vi "DS11202Z CHx-Config.vi"(0 "TestIndex":i32, 1 "通道":enum16{"Channel_1", "Channel_2"}(ring), 2 "通道开关":enum16{"ON", "OFF"}(ring), 3 "耦合":enum16{"直流", "交流", "接地"}(ring)=enum."接地", 4 "探头":enum16{"1X", "10X"}(ring)=enum."10X", 5 "幅值":dbl=1.0) -> (14 "OK?":bool, 19 "错误输出":errorcluster)   [LabVIEW 2015]
panel:
  out "Command":string
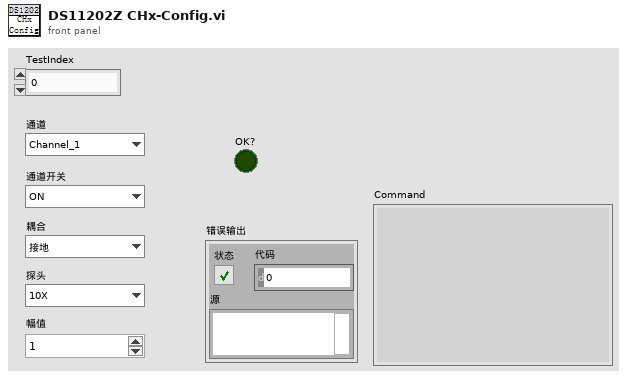
[diagram p1: front panel]
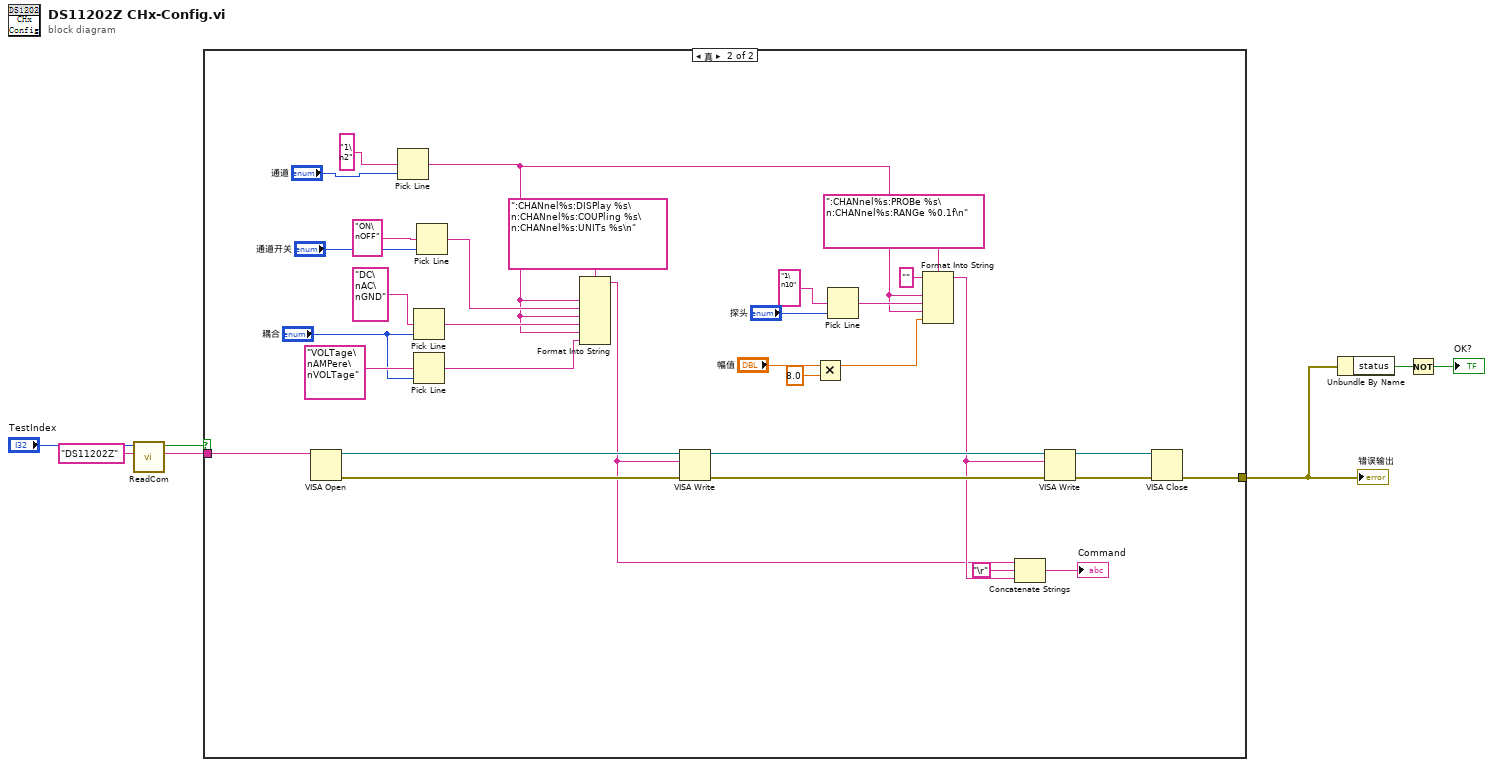
[diagram p0: block diagram]
diagram:
  n1 = call "ReadCom.vi"("仪器名称"="DS11202Z", "MyIndex"="TestIndex") -> ("COM"=w1:string, "OK?"=w2:bool)  [unwired: 7 in, 1 out]
  n2 = case shown="真" w2 {
    tunnel: [_ w34] -> w7
    tunnel: w1 -> [_ w8]
    frame False {
    }
    frame True {
      n3 = VISA Open(VISA resource name=w8) -> (VISA resource name=w39:refnum<visa-resource-name>, error out=w38:errorcluster)  [unwired: 1 in, 3 out]
      n4 = Pick Line(multi-line string="1\n2", line index="通道") -> (output string=w14:string)  [unwired: 1 in]
      n5 = Pick Line(multi-line string="DC\nAC\nGND", line index="耦合") -> (output string=w26:string)  [unwired: 1 in]
      n6 = Pick Line(multi-line string="VOLTage\nAMPere\nVOLTage", line index="耦合") -> (output string=w19:string)  [unwired: 1 in]
      n7 = Pick Line(multi-line string="ON\nOFF", line index="通道开关") -> (output string=w27:string)  [unwired: 1 in]
      n8 = Format Into String(format string=":CHANnel%s:DISPlay %s\n:CHANnel%s:COUPling %s\n:CHANnel%s:UNITs %s\n" ("字符串"), w14, w27, w14, w26, w14, w19) -> (resulting string=w10:string)  [unwired: 2 in, 1 out]
      n9 = VISA Write(VISA resource name=w39, write buffer=w10, error in (no error)=w38) -> (VISA resource name out=w37:refnum<visa-resource-name>, error out=w36:errorcluster)  [unwired: 1 out]
      n10 = Multiply(x="幅值", y=8.0) -> (x*y=w13:dbl)
      n11 = Pick Line(multi-line string="1\n10", line index="探头") -> (output string=w18:string)  [unwired: 1 in]
      n12 = Format Into String(format string=":CHANnel%s:PROBe %s\n:CHANnel%s:RANGe %0.1f\n" ("字符串"), initial string="" ("初始字符串"), w14, w18, w14, w13) -> (resulting string=w35:string)  [unwired: 1 in, 1 out]
      n13 = Concatenate Strings(w10, "\r", w35) -> (→"Command":string)
      n14 = VISA Write(VISA resource name=w37, write buffer=w35, error in (no error)=w36) -> (VISA resource name out=w23:refnum<visa-resource-name>, error out=w22:errorcluster)  [unwired: 1 out]
      n15 = VISA Close(VISA resource name=w23, error in (no error)=w22) -> (error out=w34:errorcluster)
    }
  }
  "错误输出" <- w7
  n16 = Unbundle By Name(w7) -> ("status"=w6:bool)
  n17 = Not(x=w6) -> (.not. x?=→"OK?":bool)
